vi "New_camera_snap_testcode.vi"(0 "Cam1":T2, 1 "Framerate":i32, 2 "Exposure time":dbl, 5 "CAM1 Model":enum16{"a2A5328-15ucBAS", "acA1920-155uc"}(ring), 7 "Cam2":T2, 9 "CAM2 Model":enum16{"a2A5328-15ucBAS", "acA1920-155uc"}(ring), 11 "error in (no error)":errorcluster) -> (4 "Image 1":T1(plugin-control), 6 "Image 2":T1(plugin-control), 10 "error out":errorcluster, 15 "error out 2":errorcluster)   [LabVIEW 2024]
uses:
  <vilib>/vision/driver/IMAQdx.llb/IMAQdx Acquisition Mode.ctl
  <vilib>/userDefined/High Color/IMAQdx.ctl
  Camera_ID.ctl
  <vilib>/vision/driver/IMAQdx.llb/IMAQdx Buffer Number Mode.ctl
  <vilib>/vision/driver/NI_Vision_Acquisition_Software.lvlib
panel:
  out "Cal1":path
  out "Cal2":path
  in  "Continuous?":T3
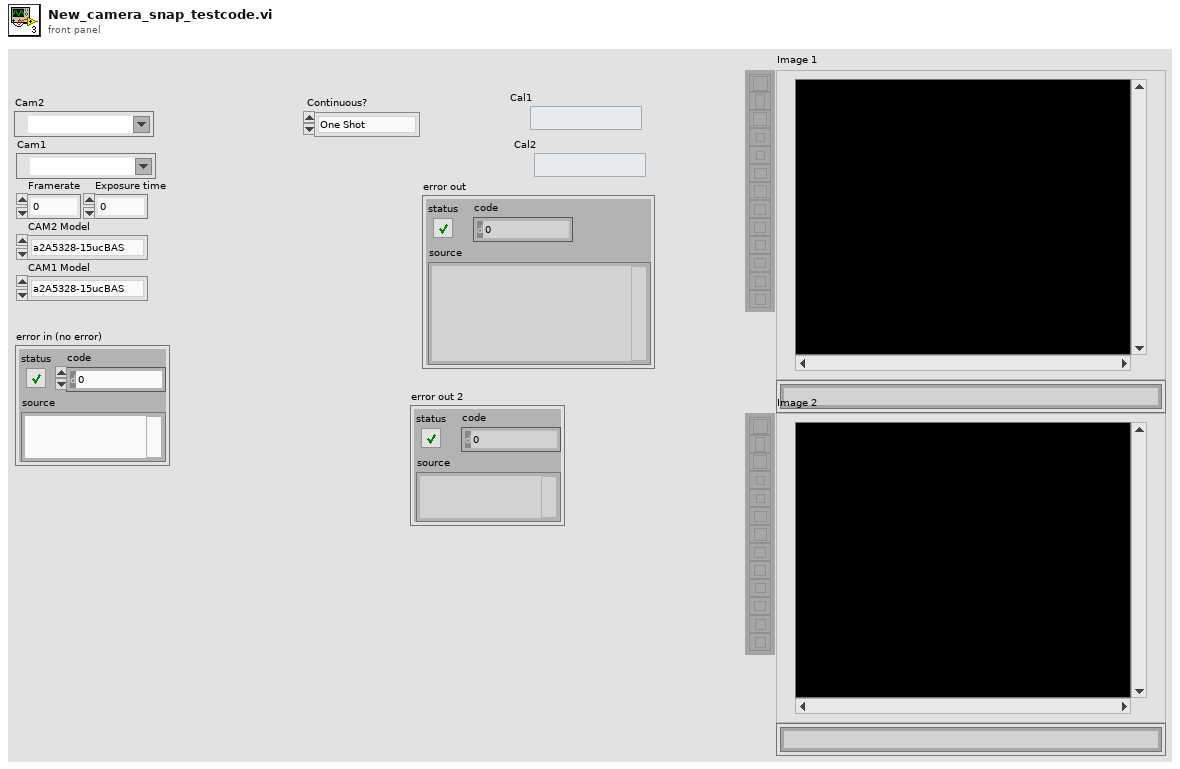
[diagram p1: front panel]
types:
  T1 = typedef "IMAQ Image.ctl" = refnum<image>
  T2 = typedef "IMAQdx.ctl" = refnum<k21>
  T3 = typedef "NI_Vision_Acquisition_Software.lvlib/IMAQdx Acquisition Mode.ctl" = enum32{"One Shot", "Continuous"}
  T4 = typedef "Camera_ID.ctl" = enum16{"Camera 1", "Camera 2"}
  T5 = typedef "NI_Vision_Acquisition_Software.lvlib/IMAQdx Buffer Number Mode.ctl" = enum32{"Next", "Last", "Buffer Number", "Every", "Last New"}
  T6 = typedef "Image Type" = u32
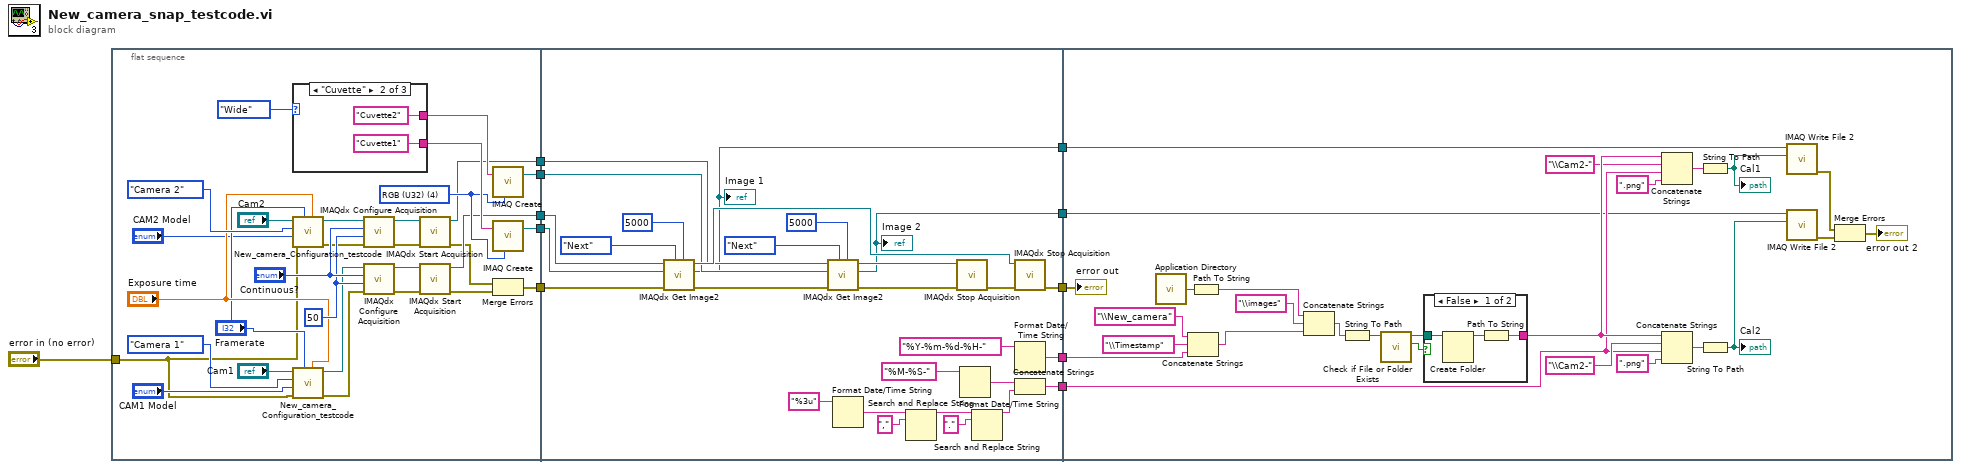
[diagram p0: block diagram]
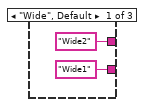
[diagram p2: hidden frame]
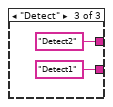
[diagram p3: hidden frame]
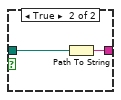
[diagram p4: hidden frame]
diagram:
  n1 = flat-sequence {
    tunnel: [w19] -> w11
    tunnel: [w18] -> w10
    tunnel: [w17] -> w9
    tunnel: [w16] -> w8
    tunnel: [w13] -> w7
    tunnel: "error in (no error)" -> [w12]
    tunnel: w11 -> [w66]
    tunnel: w10 -> [w65]
    tunnel: w9 -> [w64]
    tunnel: w8 -> [w63]
    tunnel: w7 -> [w62]
    tunnel: [w61] -> w6
    tunnel: [w52] -> w5
    tunnel: [w50] -> w4
    tunnel: [w49] -> w3
    tunnel: [w48] -> w2
    tunnel: w6 -> [w77]
    tunnel: w5 -> [w84]
    tunnel: w4 -> [w89]
    tunnel: w3 -> [w79]
    tunnel: w2 -> [w78]
    frame #0 {
      w36 = u32 50 ("Number of Buffers")
      w38 = T6 4 items=["Grayscale (U8)", "Grayscale (I16)", "Grayscale (SGL)", "Complex (CSG)", "RGB (U32)", "HSL (U32)", "RGB (U64)", "Grayscale (U16)"] ("Image Type")
      n2 = case shown="\"Cuvette\"" enum16{"Wide", "Cuvette", "Detect"}."Wide" {
        tunnel: ["Wide1" "Cuvette1" "Detect1"] -> w40
        tunnel: ["Wide2" "Cuvette2" "Detect2"] -> w39
        frame "Wide", Default {
        }
        frame "Cuvette" {
        }
        frame "Detect" {
        }
      }
      n3 = call "New_camera_Configuration_testcode.vi"("Exposure time"="Exposure time", "Framerate"="Framerate", "error in (no error)"=w12, "CAM Model"="CAM2 Model", "Camera"=Camera_ID."Camera 2", "Refnum in"="Cam2") -> ("error out 2"=w29:errorcluster, "Refnum out 2"=w28:T2)  [unwired: 4 in]
      n4 = call "New_camera_Configuration_testcode.vi"("Exposure time"="Exposure time", "Framerate"="Framerate", "error in (no error)"=w12, "CAM Model"="CAM1 Model", "Camera"=Camera_ID."Camera 1", "Refnum in"="Cam1") -> ("error out 2"=w30:errorcluster, "Refnum out 2"=w31:T2)  [unwired: 4 in]
      n5 = call <vilib>:"IMAQdx Configure Acquisition.vi"("error in"=w29, "Number of Buffers"=w36, "Continuous?"="Continuous?", "Session In"=w28) -> ("error out"=w34:errorcluster, "Session Out"=w35:T2)  [unwired: 6 in]
      n6 = call <vilib>:"IMAQdx Configure Acquisition.vi"("error in"=w30, "Number of Buffers"=w36, "Continuous?"="Continuous?", "Session In"=w31) -> ("error out"=w32:errorcluster, "Session Out"=w33:T2)  [unwired: 6 in]
      n7 = call <vilib>:"IMAQdx Start Acquisition.vi"("error in"=w34, "Session In"=w35) -> ("error out"=w14:errorcluster, "Session Out"=w18:T2)  [unwired: 8 in]
      n8 = call <vilib>:"IMAQdx Start Acquisition.vi"("error in"=w32, "Session In"=w33) -> ("error out"=w15:errorcluster, "Session Out"=w19:T2)  [unwired: 8 in]
      n9 = call "IMAQ Create"("Image Name"=w39, "Image Type"=w38) -> ("New Image"=w16:T1)  [unwired: 3 in, 1 out]
      n10 = call "IMAQ Create"("Image Name"=w40, "Image Type"=w38) -> ("New Image"=w17:T1)  [unwired: 3 in, 1 out]
      n11 = Merge Errors(w14, w15) -> (w13:errorcluster)
    }
    frame #1 {
      n12 = call <vilib>:"IMAQdx Get Image2.vi"("Timeout (ms)"=5000, "Buffer Number Mode (Next)"=IMAQdx_Buffer_Number_Mode."Next", "error in"=w62, "Image In"=w64, "Session In"=w66) -> ("error out"=w68:errorcluster, "Image Out"=w48:T1, "Session Out"=w74:T2)  [unwired: 3 in, 1 out]
      "Image 1" <- w48
      n13 = call <vilib>:"IMAQdx Get Image2.vi"("Timeout (ms)"=5000, "Buffer Number Mode (Next)"=IMAQdx_Buffer_Number_Mode."Next", "error in"=w68, "Image In"=w63, "Session In"=w65) -> ("error out"=w69:errorcluster, "Image Out"=w49:T1, "Session Out"=w75:T2)  [unwired: 3 in, 1 out]
      "Image 2" <- w49
      n14 = Format Date/Time String(time format string (%c)="%3u") -> (date/time string=w60:string)  [unwired: 2 in]
      n15 = Search and Replace String(input string=w60, search string=",") -> (result string=w54:string)  [unwired: 6 in, 3 out]
      n16 = call <vilib>:"IMAQdx Stop Acquisition.vi"("error in"=w69, "Session In"=w75) -> ("error out"=w67:errorcluster)  [unwired: 8 in, 1 out]
      n17 = Format Date/Time String(time format string (%c)="%M-%S-") -> (date/time string=w59:string)  [unwired: 2 in]
      n18 = Search and Replace String(input string=w54, search string=".") -> (result string=w53:string)  [unwired: 6 in, 3 out]
      n19 = call <vilib>:"IMAQdx Stop Acquisition.vi"("error in"=w67, "Session In"=w74) -> ("error out"=w61:errorcluster)  [unwired: 8 in, 1 out]
      n20 = Format Date/Time String(time format string (%c)="%Y-%m-%d-%H-") -> (date/time string=w50:string)  [unwired: 2 in]
      n21 = Concatenate Strings(w59, w53) -> (w52:string)
    }
    frame #2 {
      n22 = call <vilib>:"Application Directory.vi"() -> ("Application Directory"=w99:path)
      n23 = Concatenate Strings("\\New_camera" ("string"), "\\Timestamp" ("string"), w89) -> (w76:string)
      n24 = Path To String(path=w99) -> (string=w94:string)
      n25 = Concatenate Strings(w94, "\\images" ("string"), w76) -> (w92:string)
      n26 = String To Path(string=w92) -> (path=w100:path)
      n27 = call <vilib>:"Check if File or Folder Exists.vi"("path"=w100) -> ("file or folder exists?"=w102:bool, "dup path"=w101:path)  [unwired: 8 in, 1 out]
      n28 = case shown="False" w102 {
        tunnel: w101 -> [w105 w107]
        tunnel: [w103 w106] -> w86
        frame False {
          n29 = Create Folder(path (use dialog)=w105) -> (created path=w104:path)  [unwired: 2 in, 2 out]
          n30 = Path To String(path=w104) -> (string=w103:string)
        }
        frame True {
          n31 = Path To String(path=w107) -> (string=w106:string)
        }
      }
      n32 = Concatenate Strings(w86, "\\Cam2-" ("string"), w84, ".png" ("string")) -> (w83:string)
      n33 = Concatenate Strings(w86, "\\Cam2-" ("string"), w84, ".png" ("string")) -> (w97:string)
      n34 = String To Path(string=w83) -> (path=w96:path)
      "Cal1" <- w96
      n35 = String To Path(string=w97) -> (path=w95:path)
      "Cal2" <- w95
      n36 = call-poly "IMAQ Write File 2"("File Path"=w96, "Image"=w78) -> ("error out"=w82:errorcluster)  [unwired: 8 in, 1 out]
      n37 = call-poly "IMAQ Write File 2"("File Path"=w95, "Image"=w79) -> ("error out"=w81:errorcluster)  [unwired: 8 in, 1 out]
      n38 = Merge Errors(w82, w81) -> (→"error out 2":errorcluster)
      "error out" <- w77
    }
  }
